vi "PID_UPS.vi"() -> ()   [LabVIEW 2021]
uses:
  <vilib>/Instr/_visa.llb/VISA Configure Serial Port (Instr).vi
  <vilib>/ptbypt/NI_PtbyPt.lvlib
panel:
  out "PIN 3 PWM":i32
  out "A0":i32
  in  "Td":dbl=0.2
  in  "Ti":dbl=0.4
  in  "kp":dbl=0.45
  out "error":i32
  out "ERROR":dbl(slide) scale=-5.0..5.0
  in  "Com Serial":refnum<visa-resource-name>
  in  "STEP":dbl(slide) scale=0.0..100.0
  out "Waveform Chart":dynamicdata(graph)
  in  "T":dbl=0.012
  in  "OFF":bool
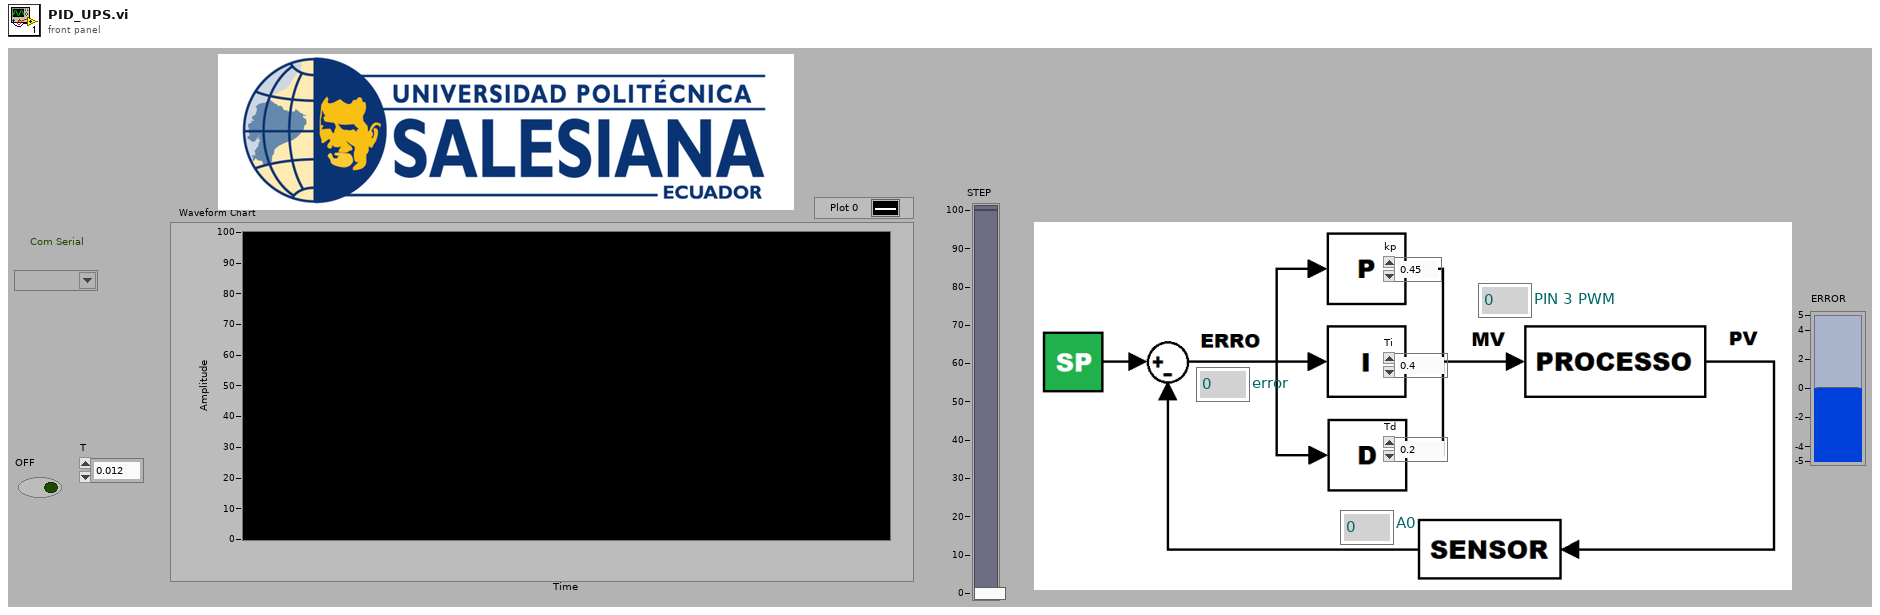
[diagram p1: front panel]
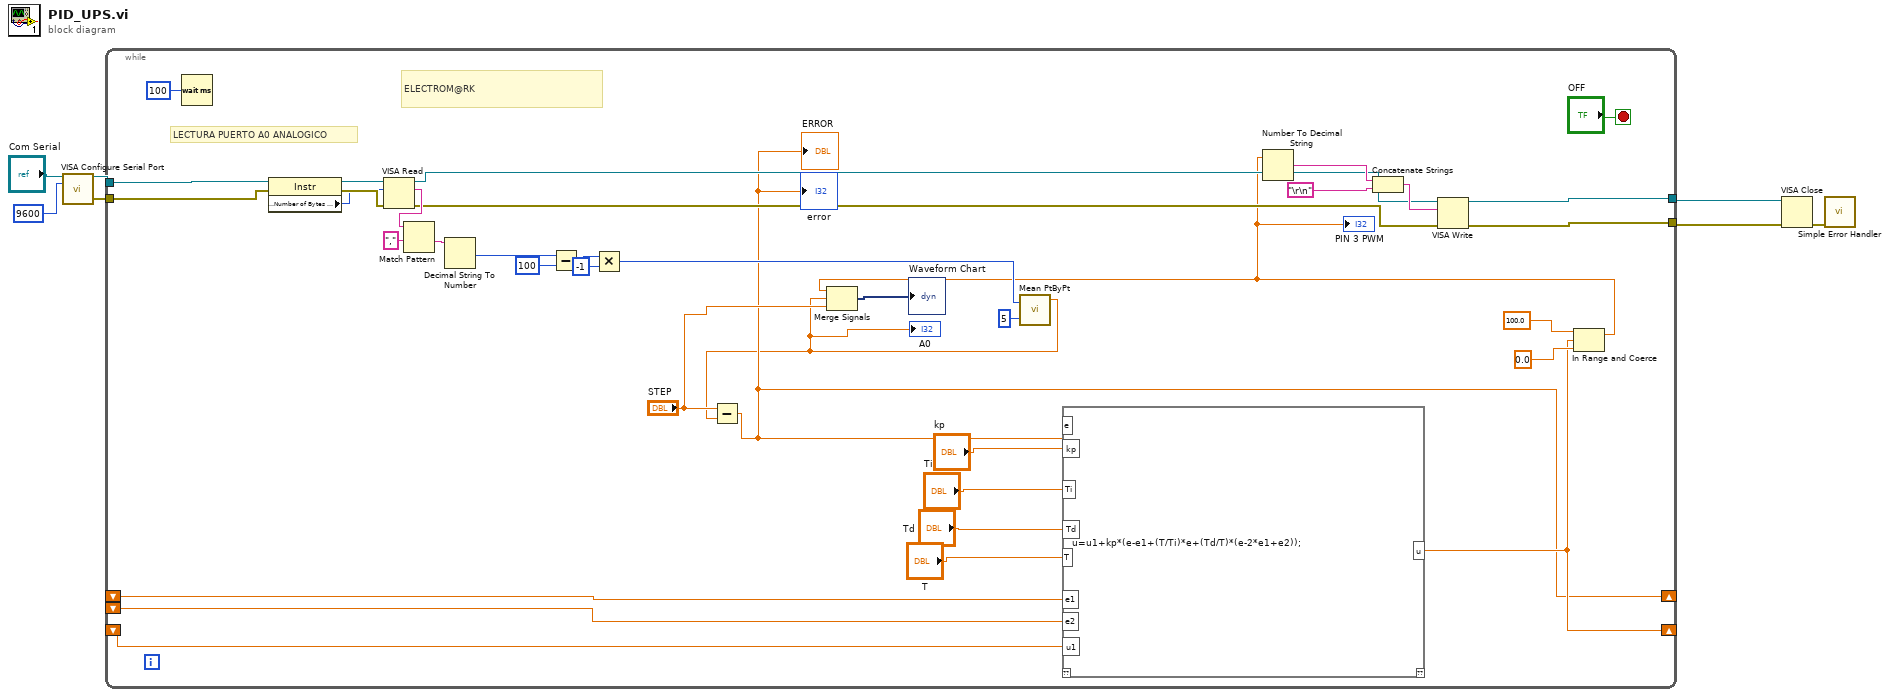
[diagram p0: block diagram]
diagram:
  n1 = call-poly "VISA Configure Serial Port"("VISA resource name"="Com Serial", "baud rate (9600)"=u32 9600) -> ("VISA resource name out"=w5:refnum<visa-resource-name>, "error out"=w4:errorcluster)  [unwired: 12 in]
  n2 = while {
    shift-right: [w21] -> _
    shift-left: _ -> [w45]
    shift-right: [w13] -> _
    shift-left: _ -> [w44]
    shift-left: _ -> [w43]
    tunnel: w5 -> [w25]
    tunnel: w4 -> [w24]
    tunnel: [w23] -> w2
    tunnel: [w22] -> w1
    stop <- "OFF" stop-if-true
    # "ELECTROM@RK"
    # "LECTURA PUERTO A0 ANALOGICO"
    n3 = Wait (ms)(milliseconds to wait=u32 100) -> ()  [unwired: 1 out]
    n4 = property class="Instr"(reference=w25, error in=w24) -> (reference out=w37:refnum<visa-resource-name>, error out=w36:errorcluster, "Serial Settings:Number of Bytes at Serial Port"=w35:u32)
    n5 = VISA Read(VISA resource name=w37, byte count=w35, error in (no error)=w36) -> (VISA resource name out=w28:refnum<visa-resource-name>, read buffer=w34:string, error out=w27:errorcluster)  [unwired: 1 out]
    n6 = Match Pattern(string=w34, regular expression=",") -> (after substring=w32:string)  [unwired: 1 in, 3 out]
    n7 = Decimal String To Number(string=w32) -> (number=w16:i32)  [unwired: 2 in, 1 out]
    n8 = Subtract(x=w16, y=100) -> (x-y=w18:i32)
    n9 = Multiply(x=w18, y=-1) -> (x*y=w14:i32)
    n10 = call <vilib>:"Mean PtByPt.vi"("x"=w14, "sample length"=5) -> ("mean"=w9:dbl)  [unwired: 2 in, 1 out]
    "A0" <- w9
    n11 = Subtract(x="STEP", y=w9) -> (x-y=w13:dbl)
    "ERROR" <- w13
    "error" <- w13
    n12 = script code="u=u1+kp*(e-e1+(T/Ti)*e+(Td/T)*(e-2*e1+e2));"("kp"="kp", "Ti"="Ti", "Td"="Td", "T"="T", "e2"=w43, "e"=w13, "u1"=w45, "e1"=w44) -> ("u"=w21:dbl)  [unwired: 1 in, 1 out]
    n13 = In Range and Coerce(upper limit=100.0, x=w21, lower limit=0.0) -> (coerced(x)=w8:dbl)  [unwired: 1 out]
    "PIN 3 PWM" <- w8
    n14 = Merge Signals(w8, w9, "STEP") -> (→"Waveform Chart":dynamicdata)
    n15 = Number To Decimal String(number=w8) -> (decimal integer string=w30:string)  [unwired: 1 in]
    n16 = Concatenate Strings(w30, "\r\n") -> (w31:string)
    n17 = VISA Write(VISA resource name=w28, write buffer=w31, error in (no error)=w27) -> (VISA resource name out=w23:refnum<visa-resource-name>, error out=w22:errorcluster)  [unwired: 1 out]
  }
  n18 = VISA Close(VISA resource name=w2, error in (no error)=w1) -> (error out=w3:errorcluster)
  n19 = call <vilib>:"Simple Error Handler.vi"("error in (no error)"=w3) -> ()  [unwired: 4 in, 5 out]
